vi "Table Save-Recall Setup.vi"(6 "Memory Location":path, 7 "Loss Compensation Type (0: Before)":u16(ring) items=["Before", "After"], 8 "error in (no error)":errorcluster, 9 "Table Type (0: Measurement ENR)":u16(ring) items=["Measurement ENR", "Calibration ENR", "Frequency", "Loss Compensation"], 10 "Operation (0:Save Table)":u16(ring) items=["Save Table", "Recall Table"], 11 "VISA resource name":refnum<visa-resource-name>) -> (0 "error out":errorcluster, 3 "VISA resource name out":refnum<visa-resource-name>)   [LabVIEW 2014, in "Agilent ESA PSA Series.lvlib"]
doc: "Saves or restores tables to or from the device storage.\n\n<B>Note:</B>\n\nThis VI is only valid in Noise Figure personality. Use <B>Switch Personality</B> VI to switch to Noise Figure before calling this VI."
uses:
  Agilent ESA PSA Series.lvlib
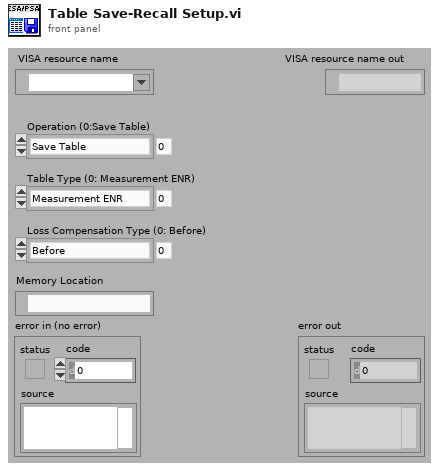
[diagram p1: front panel]
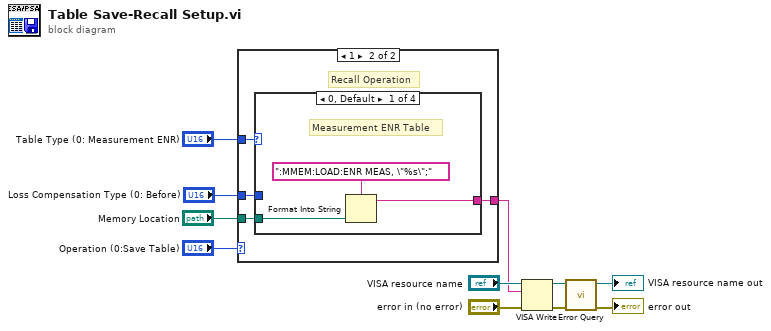
[diagram p0: block diagram]
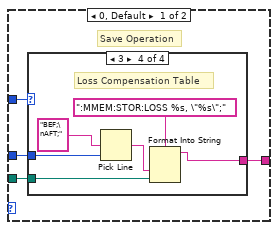
[diagram p2: hidden frame]
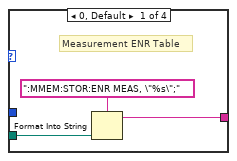
[diagram p3: hidden frame]
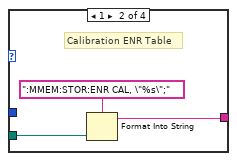
[diagram p4: hidden frame]
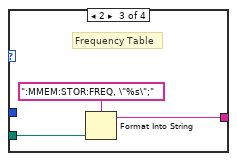
[diagram p5: hidden frame]
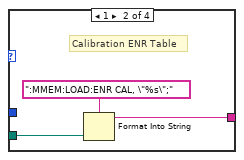
[diagram p6: hidden frame]
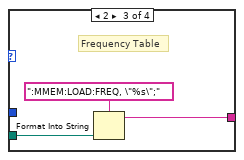
[diagram p7: hidden frame]
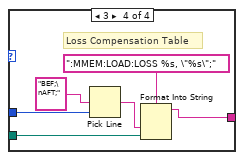
[diagram p8: hidden frame]
diagram:
  n1 = case shown="1" "Operation (0:Save Table)" {
    tunnel: "Memory Location" -> [w14 w32]
    tunnel: [w13 w34] -> w3
    tunnel: "Table Type (0: Measurement ENR)" -> [w15 w31]
    tunnel: "Loss Compensation Type (0: Before)" -> [w12 w33]
    frame 0, Default {
      # "Save Operation"
      n2 = case shown="3" w15 {
        tunnel: w14 -> [w16 w20 w24 w25]
        tunnel: [w18 w19 w22 w29] -> w13
        tunnel: w12 -> [_ _ _ w28]
        frame 0, Default {
          # "Measurement ENR Table"
          n3 = Format Into String(format string=":MMEM:STOR:ENR MEAS, \"%s\";", w16) -> (resulting string=w18:string)  [unwired: 2 in, 1 out]
        }
        frame 1 {
          # "Calibration ENR Table"
          n4 = Format Into String(format string=":MMEM:STOR:ENR CAL, \"%s\";", w20) -> (resulting string=w19:string)  [unwired: 2 in, 1 out]
        }
        frame 2 {
          # "Frequency Table"
          n5 = Format Into String(format string=":MMEM:STOR:FREQ, \"%s\";", w24) -> (resulting string=w22:string)  [unwired: 2 in, 1 out]
        }
        frame 3 {
          # "Loss Compensation Table"
          n6 = Pick Line(multi-line string="BEF;\nAFT;", line index=w28) -> (output string=w26:string)  [unwired: 1 in]
          n7 = Format Into String(format string=":MMEM:STOR:LOSS %s, \"%s\";", w26, w25) -> (resulting string=w29:string)  [unwired: 2 in, 1 out]
        }
      }
    }
    frame 1 {
      # "Recall Operation"
      n8 = case shown="0, Default" w31 {
        tunnel: [w37 w39 w42 w48] -> w34
        tunnel: w33 -> [_ _ _ w45]
        tunnel: w32 -> [w35 w38 w41 w44]
        frame 0, Default {
          # "Measurement ENR Table"
          n9 = Format Into String(format string=":MMEM:LOAD:ENR MEAS, \"%s\";", w35) -> (resulting string=w37:string)  [unwired: 2 in, 1 out]
        }
        frame 1 {
          # "Calibration ENR Table"
          n10 = Format Into String(format string=":MMEM:LOAD:ENR CAL, \"%s\";", w38) -> (resulting string=w39:string)  [unwired: 2 in, 1 out]
        }
        frame 2 {
          # "Frequency Table"
          n11 = Format Into String(format string=":MMEM:LOAD:FREQ, \"%s\";", w41) -> (resulting string=w42:string)  [unwired: 2 in, 1 out]
        }
        frame 3 {
          # "Loss Compensation Table"
          n12 = Pick Line(multi-line string="BEF;\nAFT;", line index=w45) -> (output string=w46:string)  [unwired: 1 in]
          n13 = Format Into String(format string=":MMEM:LOAD:LOSS %s, \"%s\";", w46, w44) -> (resulting string=w48:string)  [unwired: 2 in, 1 out]
        }
      }
    }
  }
  n14 = VISA Write(VISA resource name="VISA resource name", write buffer=w3, error in (no error)="error in (no error)") -> (VISA resource name out=w5:refnum<visa-resource-name>, error out=w4:errorcluster)  [unwired: 1 out]
  n15 = call "Error Query.vi"("error in (no error)"=w4, "VISA resource name"=w5) -> ("error out"=→"error out":errorcluster, "VISA resource name out"=→"VISA resource name out":refnum<visa-resource-name>)  [unwired: 6 in, 2 out]
